vi "Set Pulse Timing.vi"(7 "Output pulse channel":T1, 8 "error in (no error)":errorcluster, 9 "Duration":dbl format="%#_6ps", 10 "Start delay":dbl format="%#_6ps", 11 "DG535 Driver in":refnum<class "DG535 Driver.lvclass">) -> (0 "error out":errorcluster, 3 "DG535 Driver out":refnum<class "DG535 Driver.lvclass">)   [LabVIEW 2020, in "DG535 Driver.lvclass"]
uses:
  DG535 Driver.lvclass
  C:/GitHub/NHMFL_Core/Libraries/Instruments/VISA Instrument/VISA Instrument.lvclass
  DG Pulse Output Channel.ctl
  VISA Instrument/VISA Instrument.lvclass/VISA Instrument.ctl
  VISA Instrument/Read VISA resource.vi
  VISA Instrument/Write VISA resource.vi
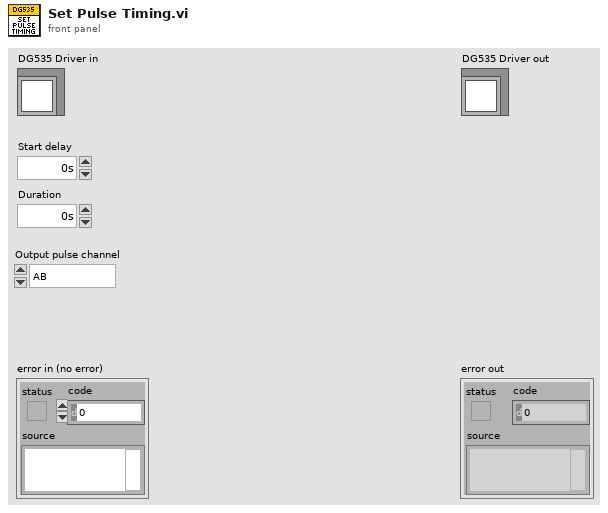
[diagram p1: front panel]
types:
  T1 = typedef "DG Pulse Output Channel.ctl" = enum16{"AB", "CD"}
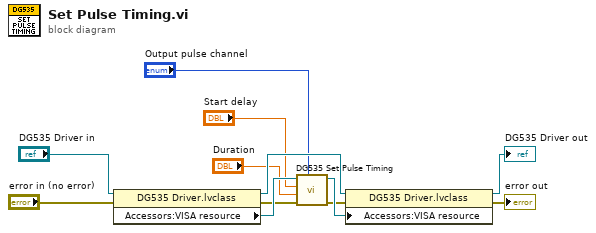
[diagram p0: block diagram]
diagram:
  n1 = property class="DG535 Driver.lvclass"(reference="DG535 Driver in", error in="error in (no error)") -> (reference out=w9:refnum<class "DG535 Driver.lvclass">, error out=w7:errorcluster, "Accessors:VISA resource"=w10:refnum<visa-resource-name>)
  n2 = call "DG535 Set Pulse Timing.vi"("Output pulse channel"="Output pulse channel", "error in"=w7, "Duration"="Duration", "Start delay"="Start delay", "VISA resource name"=w10) -> ("error out"=w5:errorcluster, "VISA resource name out"=w8:refnum<visa-resource-name>)  [unwired: 4 in, 1 out]
  n3 = property class="DG535 Driver.lvclass"(reference=w9, error in=w5, "Accessors:VISA resource"=w8) -> (reference out=→"DG535 Driver out":refnum<class "DG535 Driver.lvclass">, error out=→"error out":errorcluster)
